vi "Teardown.vi"(8 "error in (no error)":errorcluster, 11 "Configuration File Interface Test In":refnum<class "Configuration File Process Interface Test.lvclass">) -> (0 "error out":errorcluster, 3 "Configuration File Interface Test Out":refnum<class "Configuration File Process Interface Test.lvclass">)   [LabVIEW 2020, in "Configuration File Process Interface Test.lvclass"]
uses:
  Configuration File Process Interface Test.lvclass
  Configuration File Process Interface Test.lvclass/Configuration File Process Interface Test.ctl
  Mock Configurable Process/Mock Configurable Process.lvclass
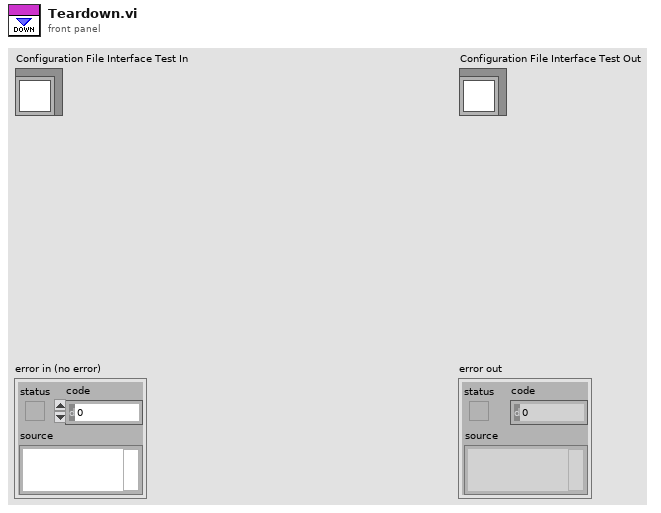
[diagram p1: front panel]
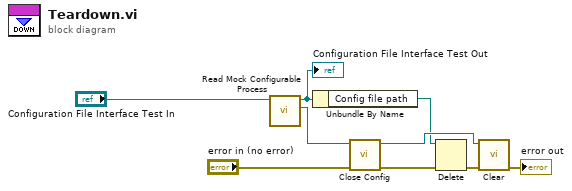
[diagram p0: block diagram]
diagram:
  n1 = call "Read Mock Configurable Process.vi"("Configuration File Process Interface Test in"="Configuration File Interface Test In") -> ("Mock Configurable.lvclass"=w3:refnum<class "Mock Configurable Process.lvclass">, "Configuration File Process Interface Test out"=w2:refnum<class "Configuration File Process Interface Test.lvclass">)  [unwired: 9 in]
  "Configuration File Interface Test Out" <- w2
  n2 = Unbundle By Name(w2) -> ("Config file path"=w1:path)
  n3 = call-dynamic "Close Config.vi"("error in (no error)"="error in (no error)", "Configuration File File In"=w3) -> ("error out"=w7:errorcluster, "Configuration File File Out"=w6:refnum<class "Mock Configurable Process.lvclass">)  [unwired: 8 in]
  n4 = Delete(path (use dialog)=w1, error in=w7) -> (error out=w8:errorcluster)  [unwired: 3 in, 2 out]
  n5 = call-dynamic "Clear.vi"("error in (no error)"=w8, "Process In"=w6) -> ("error out"=→"error out":errorcluster)  [unwired: 9 in]
